vi "Create RxTx.vi"(8 "error in (no error)":errorcluster, 11 "Channel in":refnum<class "Channel.lvclass">) -> (0 "error out":errorcluster, 3 "Channel out":refnum<class "Channel.lvclass">)   [LabVIEW 2018, in "Channel.lvclass"]
doc: "Create the queres responsible for communication"
uses:
  Channel.lvclass
  Channel.lvclass/Channel.ctl
  RxTx/CCS_RxTx.lvclass
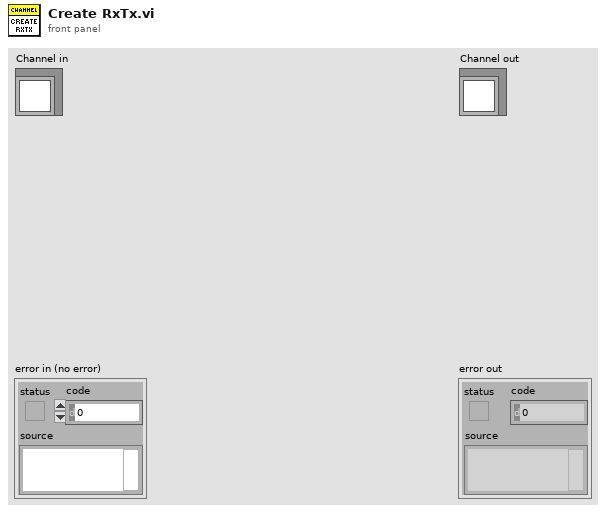
[diagram p1: front panel]
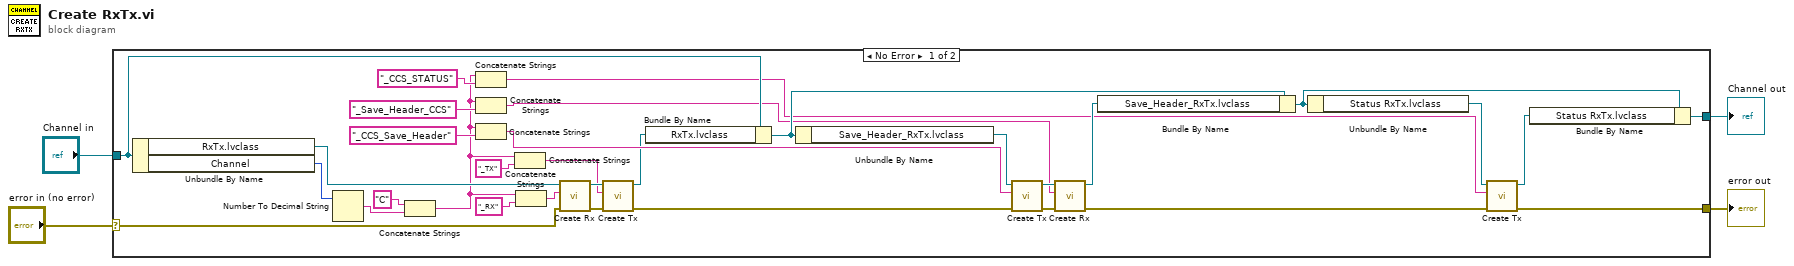
[diagram p0: block diagram]
diagram:
  n1 = case shown="No Error" "error in (no error)" {
    selector: "error in (no error)" -> [w23 w38]
    tunnel: [w6 w38] -> w3
    tunnel: [w5 w37] -> w1
    tunnel: "Channel in" -> [w33 w37]
    frame No Error {
      n2 = Unbundle By Name(w33) -> ("RxTx.lvclass"=w35:refnum<class "CCS_RxTx.lvclass">, "Channel"=w14:u8)
      n3 = Number To Decimal String(number=w14) -> (decimal integer string=w30:string)  [unwired: 1 in]
      n4 = Concatenate Strings("C", w30) -> (w8:string)
      n5 = Concatenate Strings(w8, "_CCS_STATUS") -> (w7:string)
      n6 = Concatenate Strings(w8, "_Save_Header_CCS") -> (w19:string)
      n7 = Concatenate Strings(w8, "_CCS_Save_Header") -> (w17:string)
      n8 = Concatenate Strings(w8, "_TX") -> (w28:string)
      n9 = Concatenate Strings(w8, "_RX") -> (w26:string)
      n10 = call "Create Rx.vi"("error in (no error)"=w23, "Reader Name"=w26, "RxTx in"=w35) -> ("error out"=w36:errorcluster, "RxTx out"=w34:refnum<class "CCS_RxTx.lvclass">)  [unwired: 7 in]
      n11 = call "Create Tx.vi"("error in (no error)"=w36, "Writer Name"=w28, "RxTx in"=w34) -> ("error out"=w15:errorcluster, "RxTx out"=w16:refnum<class "CCS_RxTx.lvclass">)  [unwired: 7 in]
      n12 = Bundle By Name(cluster=w33, "RxTx.lvclass"=w16) -> (w24:refnum<class "Channel.lvclass">)
      n13 = Unbundle By Name(w24) -> ("Save_Header_RxTx.lvclass"=w32:refnum<class "CCS_RxTx.lvclass">)
      n14 = call "Create Tx.vi"("error in (no error)"=w15, "Writer Name"=w17, "RxTx in"=w32) -> ("error out"=w21:errorcluster, "RxTx out"=w20:refnum<class "CCS_RxTx.lvclass">)  [unwired: 7 in]
      n15 = call "Create Rx.vi"("error in (no error)"=w21, "Reader Name"=w19, "RxTx in"=w20) -> ("error out"=w10:errorcluster, "RxTx out"=w22:refnum<class "CCS_RxTx.lvclass">)  [unwired: 7 in]
      n16 = Bundle By Name(cluster=w24, "Save_Header_RxTx.lvclass"=w22) -> (w12:refnum<class "Channel.lvclass">)
      n17 = Unbundle By Name(w12) -> ("Status RxTx.lvclass"=w13:refnum<class "CCS_RxTx.lvclass">)
      n18 = call "Create Tx.vi"("error in (no error)"=w10, "Writer Name"=w7, "RxTx in"=w13) -> ("error out"=w6:errorcluster, "RxTx out"=w11:refnum<class "CCS_RxTx.lvclass">)  [unwired: 7 in]
      n19 = Bundle By Name(cluster=w12, "Status RxTx.lvclass"=w11) -> (w5:refnum<class "Channel.lvclass">)
    }
    frame Error {
    }
  }
  "error out" <- w3
  "Channel out" <- w1
